vi "Push Button.vi"() -> ()   [LabVIEW 2022 SP3]
uses:
  <vilib>/DAQmx/read.llb/DAQmx Read (Counter U32 1Chan 1Samp).vi
  <vilib>/DAQmx/write.llb/DAQmx Write (Digital U8 1Chan 1Samp).vi
  <vilib>/DAQmx/miscellaneous.llb/DAQmx Fill In Error Info.vi
panel:
  out "Boolean Array":bool[](array[boolean])
  out "data":u32
  in  "stop":bool
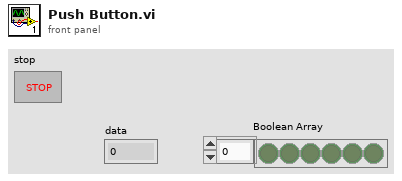
[diagram p1: front panel]
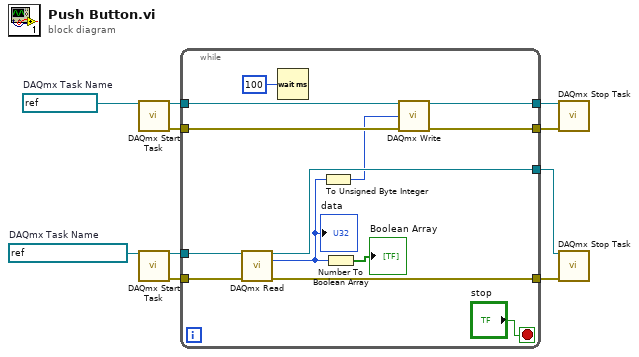
[diagram p0: block diagram]
diagram:
  w7 = refnum<k21> "LEDsPort"  # DAQmx Task Name
  w10 = refnum<k21> "Push Button CTN"  # DAQmx Task Name
  n1 = call <vilib>:"DAQmx Start Task.vi"("task/channels in"=w7) -> ("task out"=w6:refnum<k21>, "error out"=w5:errorcluster)  [unwired: 13 in]
  n2 = call <vilib>:"DAQmx Start Task.vi"("task/channels in"=w10) -> ("task out"=w9:refnum<k21>, "error out"=w4:errorcluster)  [unwired: 13 in]
  n3 = while {
    tunnel: w9 -> [w23]
    tunnel: [w22] -> w8
    tunnel: w4 -> [w18]
    tunnel: [w14] -> w1
    tunnel: w6 -> [w20]
    tunnel: [w16] -> w3
    tunnel: w5 -> [w19]
    tunnel: [w15] -> w2
    stop <- "stop" stop-if-true
    n4 = call-poly <vilib>:"DAQmx Read.vi"("task/channels in"=w23, "error in"=w18) -> ("task out"=w22:refnum<k21>, "data"=w12:u32, "error out"=w14:errorcluster)  [unwired: 11 in]
    "data" <- w12
    n5 = Wait (ms)(milliseconds to wait=100) -> ()  [unwired: 1 out]
    n6 = To Unsigned Byte Integer(number=w12) -> (unsigned 8bit integer=w11:u8)
    n7 = Number To Boolean Array(number=w12) -> (Boolean array=→"Boolean Array":bool[])
    n8 = call-poly <vilib>:"DAQmx Write.vi"("task/channels in"=w20, "data"=w11, "error in"=w19) -> ("task out"=w16:refnum<k21>, "error out"=w15:errorcluster)  [unwired: 10 in, 1 out]
  }
  n9 = call <vilib>:"DAQmx Stop Task.vi"("task/channels in"=w3, "error in"=w2) -> ()  [unwired: 12 in, 2 out]
  n10 = call <vilib>:"DAQmx Stop Task.vi"("task/channels in"=w8, "error in"=w1) -> ()  [unwired: 12 in, 2 out]
